vi "Delete.vi"(8 "error in (no error)":errorcluster, 11 "ViewerRef":T1) -> (0 "error out":errorcluster)   [LabVIEW 2018, in "TopicViewer.lvlib"]
uses:
  TopicViewer.lvlib
  controls/viewewr_bus.ctl
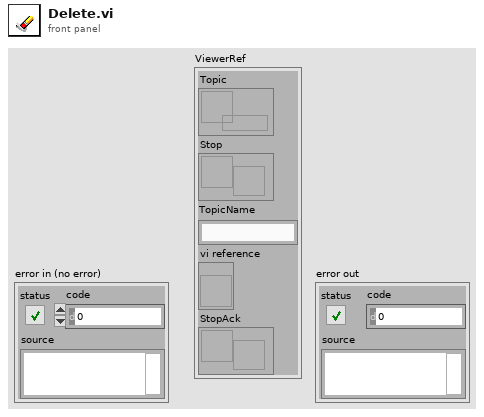
[diagram p1: front panel]
types:
  T1 = typedef "TopicViewer.lvlib/viewewr_bus.ctl" = cluster{"Topic":refnum<queue>, "Stop":refnum<notifier>, "TopicName":string, "vi reference":refnum<vi>, "StopAck":refnum<notifier>}
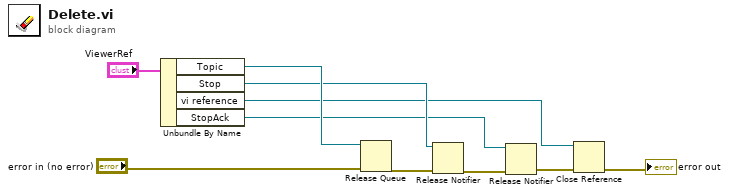
[diagram p0: block diagram]
diagram:
  n1 = Unbundle By Name("ViewerRef") -> ("Topic"=w9:refnum<queue>, "Stop"=w7:refnum<notifier>, "vi reference"=w5:refnum<vi>, "StopAck"=w6:refnum<notifier>)
  n2 = Release Queue(queue=w9, error in (no error)="error in (no error)") -> (error out=w4:errorcluster)  [unwired: 1 in, 2 out]
  n3 = Release Notifier(notifier=w7, error in (no error)=w4) -> (error out=w3:errorcluster)  [unwired: 1 in, 2 out]
  n4 = Release Notifier(notifier=w6, error in (no error)=w3) -> (error out=w2:errorcluster)  [unwired: 1 in, 2 out]
  n5 = Close Reference(reference=w5, error in (no error)=w2) -> (error out=→"error out":errorcluster)
